vi "UI Producer Consumer-generate-waveform.vi"() -> ()   [LabVIEW 2020]
doc: "This VI illustrates an architecture that allows the user to queue multiple processes. Each process contains multiple state, or in this case stages.The queueing of events is handled by the producer UI loop while the consumer loop goes through each process' states. The processes can have functionality different from one another or can have the same functionality. This architecture allows for expansion on the number of processes as well as the number of states for each process by augmenting the states enum and inputting state functionality in the state case. I have changed the consumer loop to have a time of 500 ms in order to make it easier for the user to enqueue elements. The slowed down consumer loops allowed queue processes to build due to the slow progression of the queue. To hasten the program, the user can change the time constant.\n\nThis type of architecture can apply to an application containing multiple processes, who each have multiple states. This allows the user to easily queue up processes that will proceed in the order that the user selects. There is also two different stop functionalities in order to ensure that a current process is completed or that the current state is completed before stopping the program. This can easily be scaled by editing the type-def enum and adding states to the state machine."
uses:
  States.ctl
panel:
  in  "Output Array":T1(array[cluster])=[{"Waveform Type"=0, "Amplitude"=1.0, "Frequency"=10.0}] {"Frequency" format="%0.2p"; "Amplitude" format="%0.2p"; "Waveform Type" items=["Sine Wave", "Triangle Wave", "Square Wave", "Sawtooth Wave"]}
  in  "Physical Channel(s)":tag="DAQ1/ao0"
  in  "error in (no error)":errorcluster
  out "error out":errorcluster
  in  "Emergency Stop Button":bool
  out "Queue":T2[](array[typedef])
  out "Cluster":T3
  in  "Stop Button":bool
  in  "Process 3":bool
  in  "Process 2":bool
  in  "Process 1":bool
  # "Overview: A producer/consumer architecture with a UI producer loop and a state machine consumer loop. Allows the user to queue multiple state sequences.\nRequirements: LabVIEW 2012 (or compatible\nInstructions:\n1. Run the VI.\n2. Press various Process buttons to see the Queue build.\n3. See the Process and Stage in the Cluster of Boolean indicators.\n4. Press Stop during Process to see Stop functionality.\n5. Run VI again after the program has stopped.\n6. Repeat step 2.\n7. Press Emergency Stop button to see Emergency Stop functionality."
  # "Click the Process button of your choice to enqueue the process of your choice. \nThe Processes will execute in the order that you queue them in."
  # "Stop Button stops program after current process has finished"
  # "Emergency Stop Button stops program after the current state. Press this button to stop in the middle of a Process"
  # "Shows the current Queue."
  # "The Boolean Cluster shows you what process is occurring and the stage it is on.\nEach stage corresponds to a state in a process."
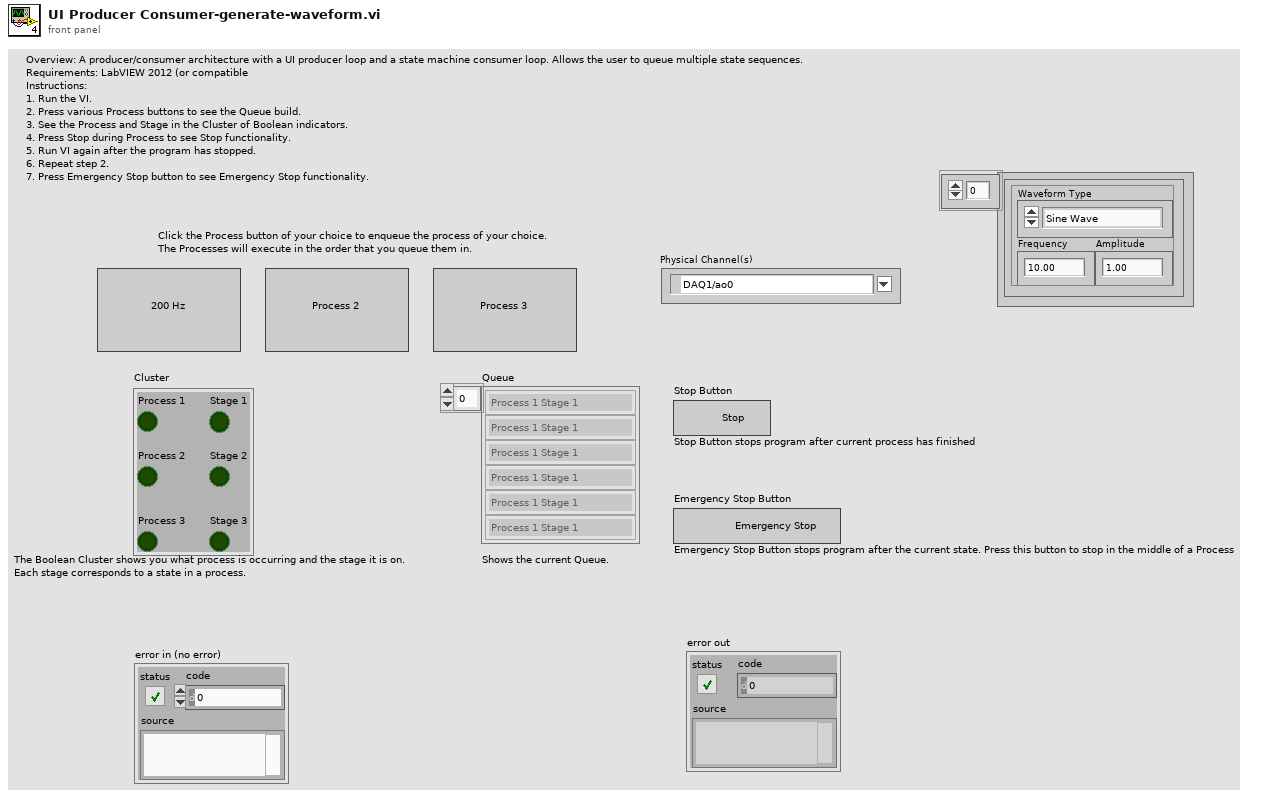
[diagram p1: front panel]
types:
  T1 = cluster{"Waveform Type":u16, "Amplitude":dbl, "Frequency":dbl}[]
  T2 = typedef "States.ctl" = enum16{"Process 1 Stage 1", "Process 1 Stage 2", "Process 1 Stage 3", "Process 2 Stage 1", "Process 2 Stage 2", "Process 2 Stage 3", "Process 3 Stage 1", "Process 3 Stage 2", "Process 3 Stage 3", "Wait", "Stop", "Emergency Stop"}
  T3 = cluster{"Process 1":bool, "Stage 1":bool, "Process 2":bool, "Stage 2":bool, "Process 3":bool, "Stage 3":bool}
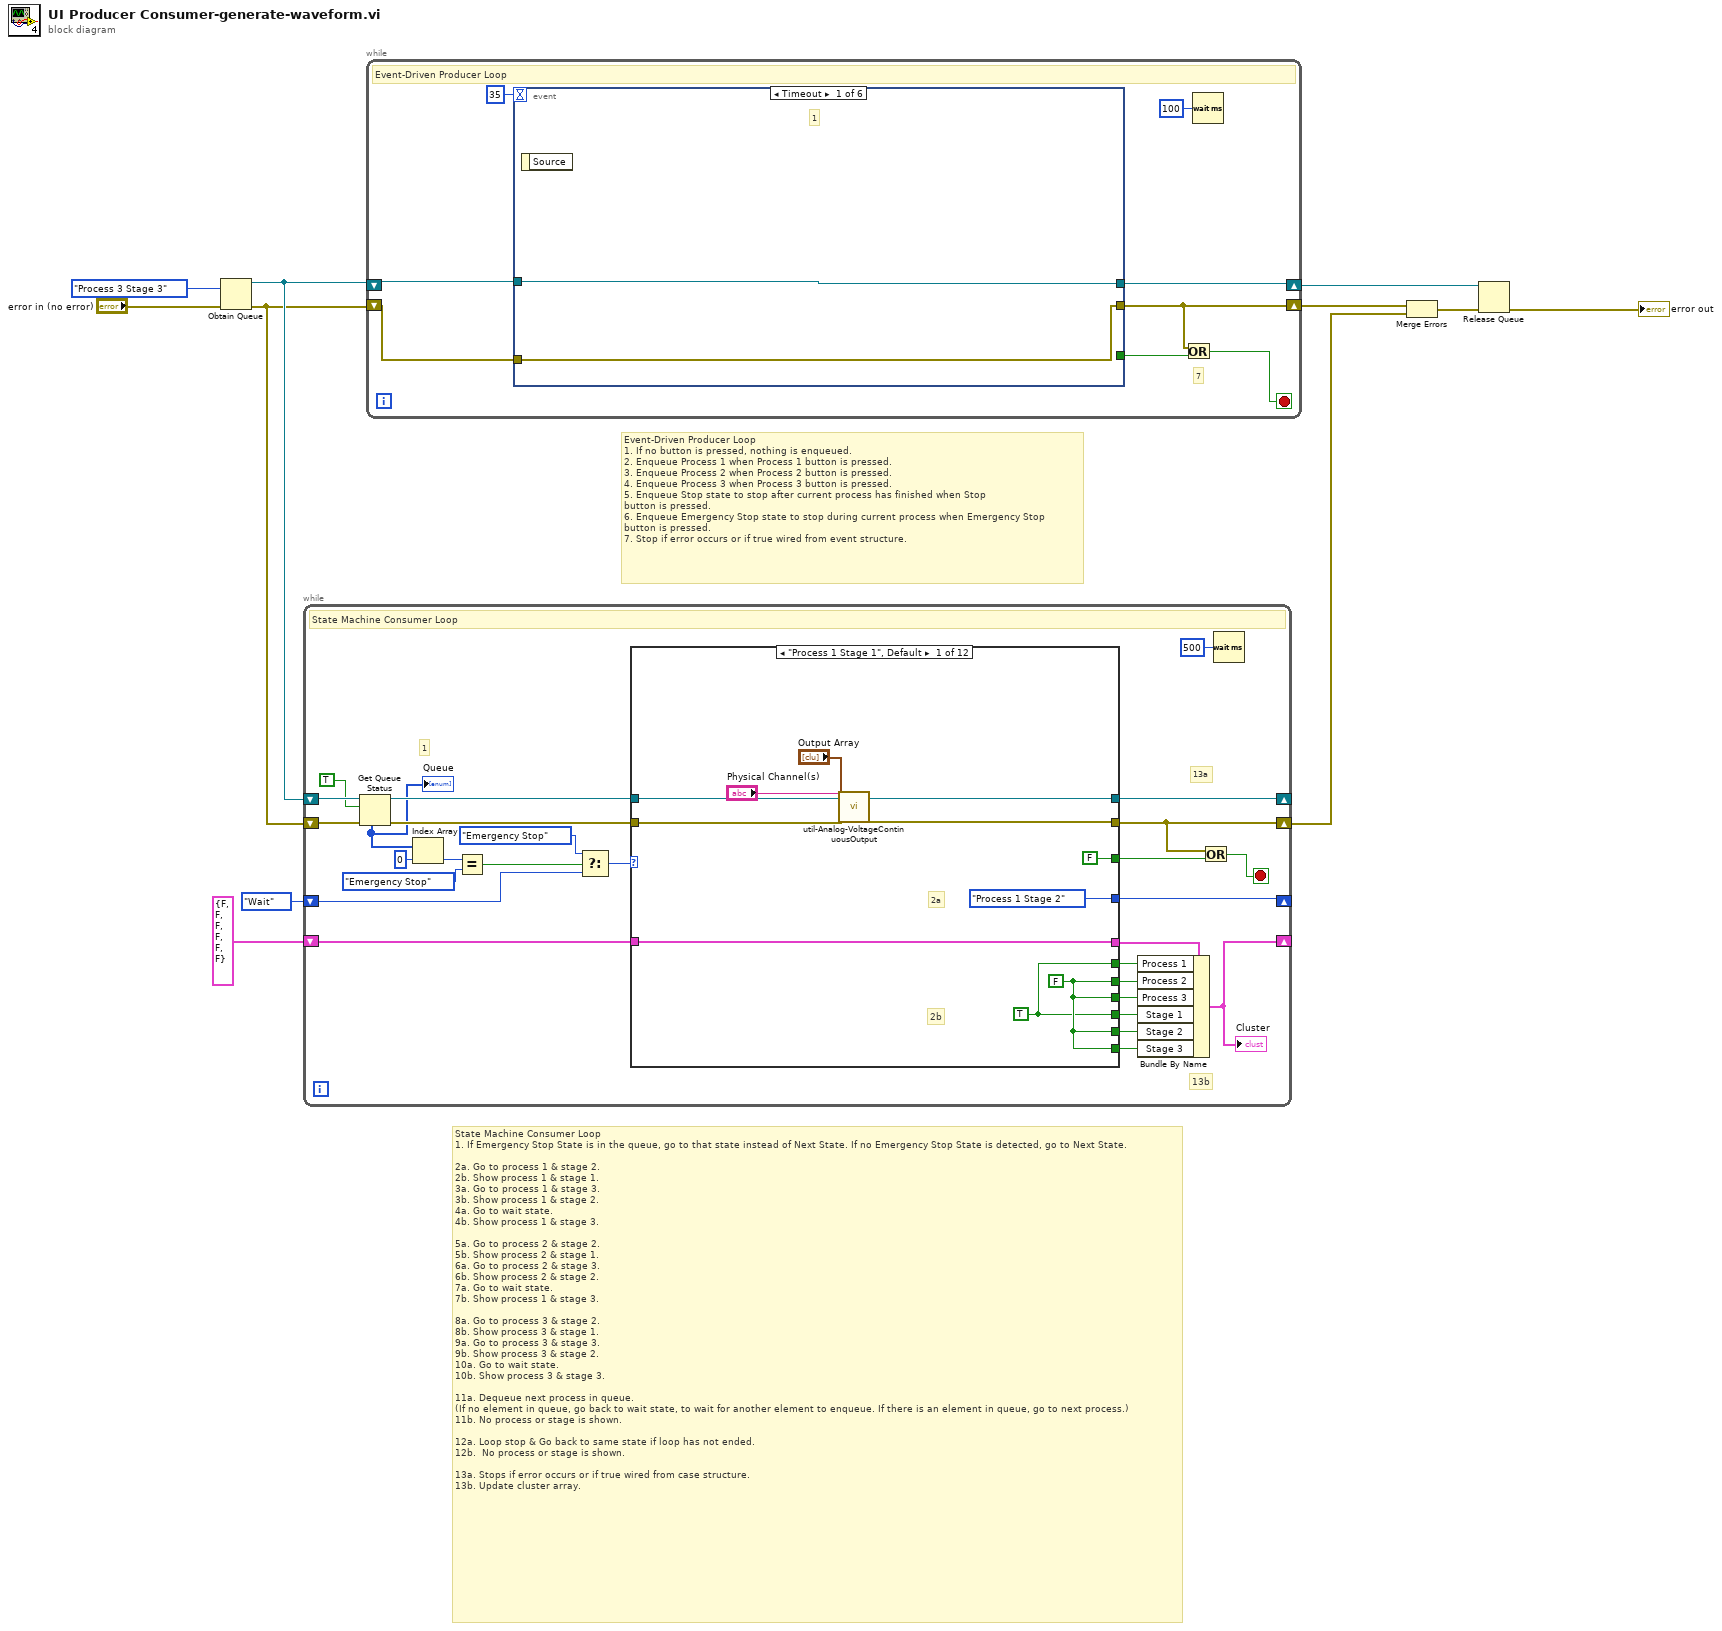
[diagram p0: block diagram]
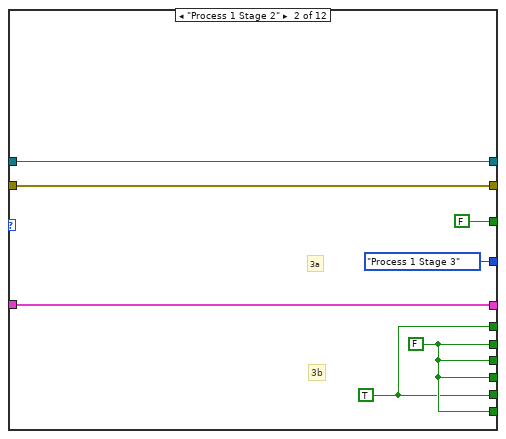
[diagram p2: hidden frame]
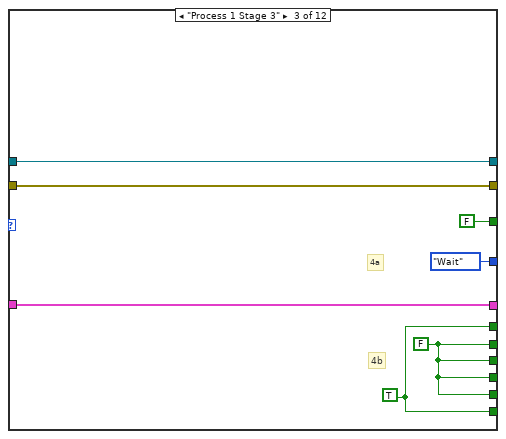
[diagram p3: hidden frame]
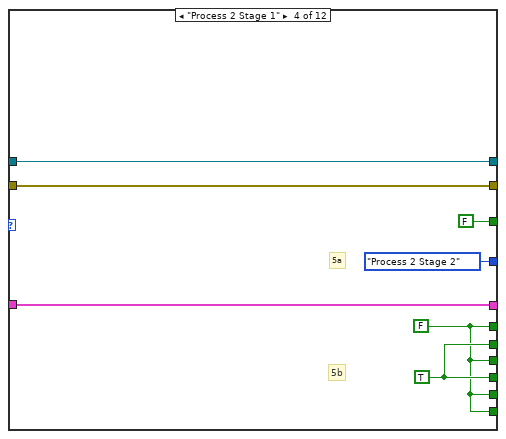
[diagram p4: hidden frame]
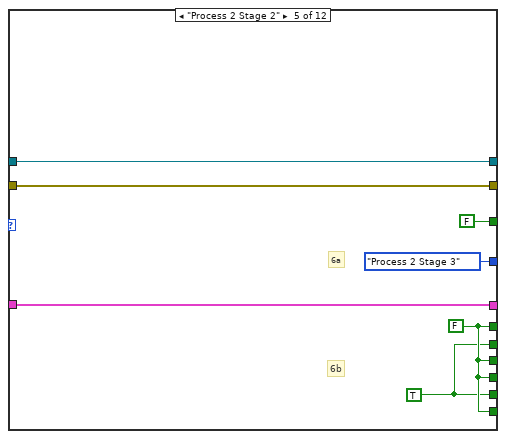
[diagram p5: hidden frame]
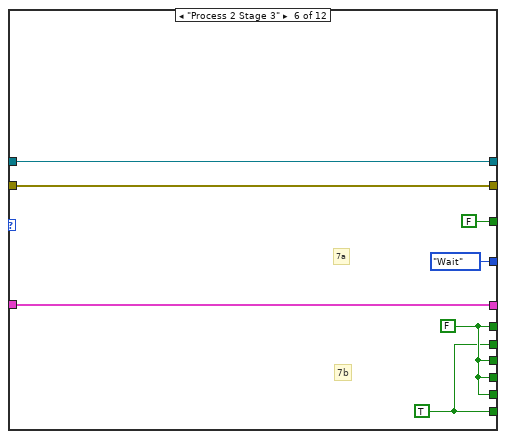
[diagram p6: hidden frame]
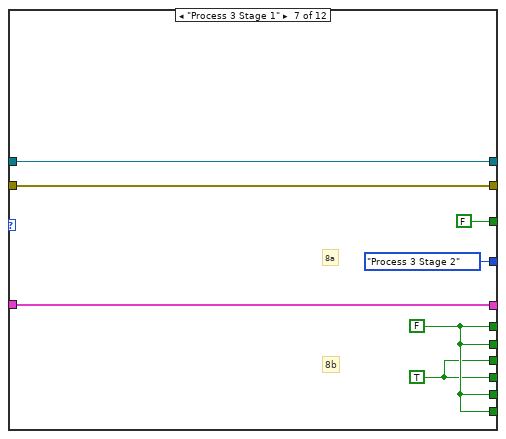
[diagram p7: hidden frame]
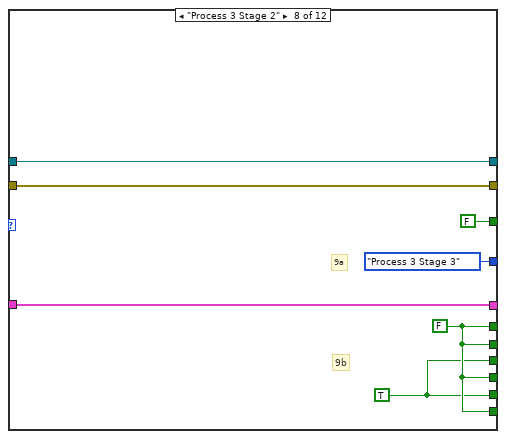
[diagram p8: hidden frame]
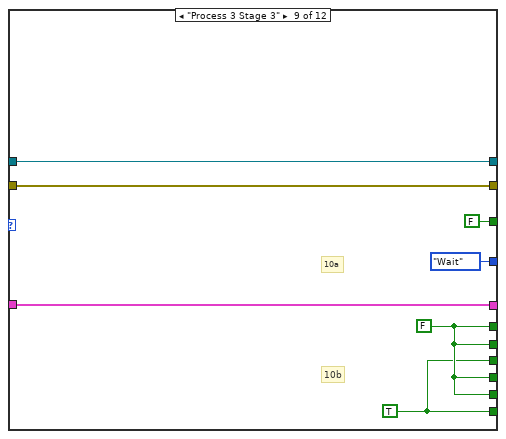
[diagram p9: hidden frame]
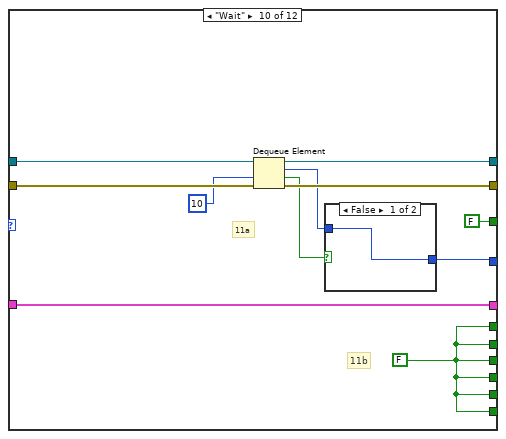
[diagram p10: hidden frame]
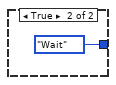
[diagram p11: hidden frame]
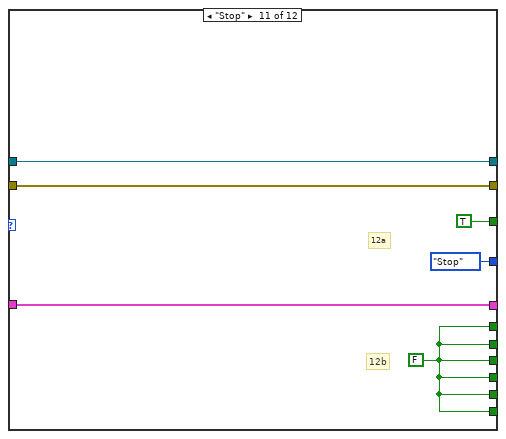
[diagram p12: hidden frame]
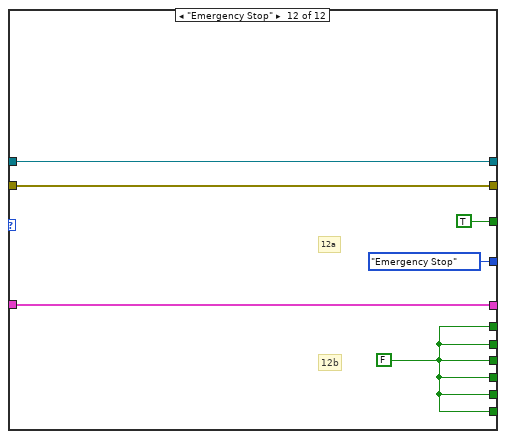
[diagram p13: hidden frame]
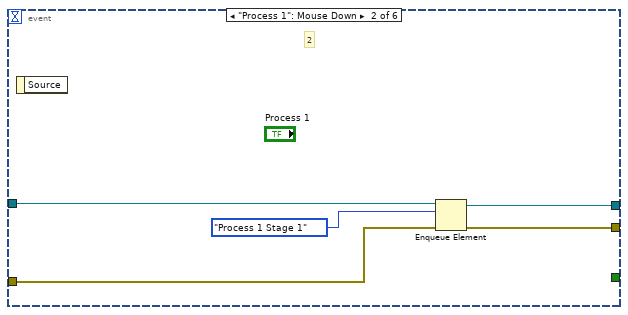
[diagram p14: hidden frame]
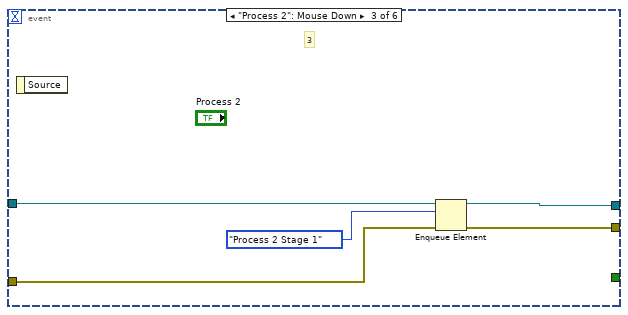
[diagram p15: hidden frame]
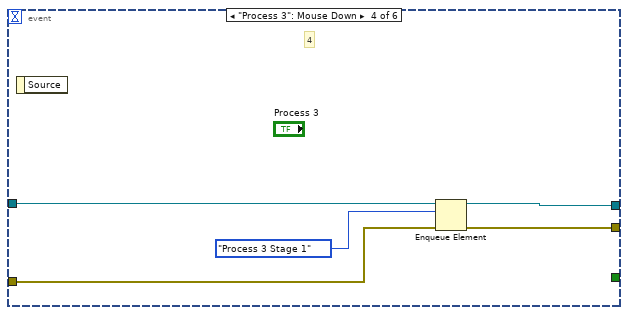
[diagram p16: hidden frame]
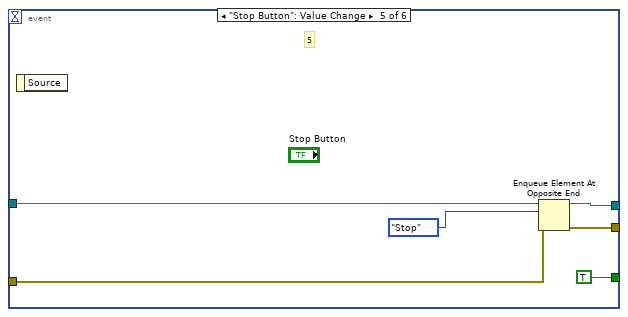
[diagram p17: hidden frame]
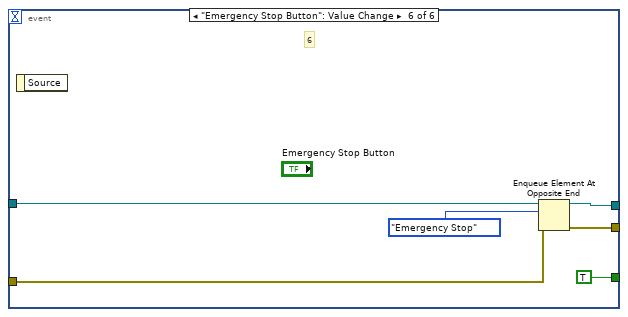
[diagram p18: hidden frame]
diagram:
  # "State Machine Consumer Loop\n1. If Emergency Stop State is in the queue, go to that state instead of Next State. If no Emergency Stop State is detected, go to Next State.\n\n2a. Go to process 1 & stage 2.\n2b. Show process 1 & stage 1.\n3a. Go to process 1 & stage 3.\n3b. Show process 1 & stage 2.\n4a. Go to wait state.\n4b. Show process 1 & stage 3.\n\n5a. Go to process 2 & stage 2.\n5b. Show process 2 & stage 1.\n6a. Go to process 2 & stage 3.\n6b. Show process 2 & stage 2.\n7a. Go to wait state.\n7b. Show process 1 & stage 3.\n\n8a. Go to process 3 & stage 2.\n8b. Show process 3 & stage 1.\n9a. Go to process 3 & stage 3.\n9b. Show process 3 & stage 2.\n10a. Go to wait state.\n10b. Show process 3 & stage 3.\n\n11a. Dequeue next process in queue.\n(If no element in queue, go back to wait state, to wait for another element to enqueue. If there is an element in queue, go to next process.)\n11b. No process or stage is shown.\n\n12a. Loop stop & Go back to same state if loop has not ended.\n12b.  No process or stage is shown.\n\n13a. Stops if error occurs or if true wired from case structure.\n13b. Update cluster array."
  # "Event-Driven Producer Loop\n1. If no button is pressed, nothing is enqueued.\n2. Enqueue Process 1 when Process 1 button is pressed.\n3. Enqueue Process 2 when Process 2 button is pressed.\n4. Enqueue Process 3 when Process 3 button is pressed.\n5. Enqueue Stop state to stop after current process has finished when Stop\nbutton is pressed.\n6. Enqueue Emergency Stop state to stop during current process when Emergency Stop\nbutton is pressed.\n7. Stop if error occurs or if true wired from event structure."
  n1 = Obtain Queue(element data type=States."Process 3 Stage 3", error in (no error)="error in (no error)") -> (queue out=w11:refnum<queue>, error out=w10:errorcluster)  [unwired: 3 in, 1 out]
  n2 = while {
    shift-right: [w25] -> _
    shift-left: w11 -> [w37]
    shift-right: [w21] -> w3
    shift-left: w10 -> [w36]
    shift-right: [w24] -> _
    shift-left: States."Wait" ("y") -> [w14]
    shift-right: [w32] -> _
    shift-left: T3 {"Process 1"=FALSE, "Stage 1"=FALSE, "Process 2"=FALSE, "Stage 2"=FALSE, "Process 3"=FALSE, "Stage 3"=FALSE} ("Cluster") -> [w34]
    stop <- w39 stop-if-true
    # "13a"
    # "13b"
    # "1"
    # "State Machine Consumer Loop"
    n3 = Get Queue Status(queue=w37, return elements? (F)=TRUE, error in (no error)=w36) -> (queue out=w35:refnum<queue>, error out=w22:errorcluster, elements=w19:T2[])  [unwired: 5 out]
    "Queue" <- w19
    n4 = Index Array(array=w19, index=0) -> (element=w17:T2)
    n5 = Equal?(x=w17, y=States."Emergency Stop") -> (x = y?=w15:bool)
    n6 = Select(t=States."Emergency Stop", s=w15, f=w14) -> (s? t:f=w12:T2)
    n7 = case shown="\"Process 1 Stage 1\", Default" w12 {
      tunnel: w35 -> [w46 w53 w62 w69 w76 w83 w90 w97 w104 w114 w124 w130]
      tunnel: w22 -> [w43 w52 w61 w68 w75 w82 w89 w96 w103 w113 w123 w129]
      tunnel: w34 -> [w49 w56 w63 w70 w77 w84 w91 w98 w105 w116 w122 w128]
      tunnel: [w49 w56 w63 w70 w77 w84 w91 w98 w105 w116 w122 w128] -> w33
      tunnel: [w47 w54 w59 w66 w74 w81 w88 w95 w102 w115 w121 w127] -> w31
      tunnel: [w48 w54 w60 w66 w73 w81 w88 w94 w102 w115 w121 w127] -> w30
      tunnel: [w48 w55 w60 w67 w73 w80 w88 w95 w102 w115 w121 w127] -> w29
      tunnel: [w48 w55 w60 w66 w74 w81 w87 w94 w101 w115 w121 w127] -> w28
      tunnel: [w47 w55 w60 w67 w74 w81 w87 w95 w102 w115 w121 w127] -> w27
      tunnel: [w48 w55 w59 w66 w74 w80 w88 w95 w101 w115 w121 w127] -> w26
      tunnel: [w46 w53 w62 w69 w76 w83 w90 w97 w104 w112 w124 w130] -> w25
      tunnel: [w42 w52 w61 w68 w75 w82 w89 w96 w103 w111 w123 w129] -> w21
      tunnel: [States."Process 1 Stage 2" ("y") States."Process 1 Stage 3" ("y") States."Wait" ("y") States."Process 2 Stage 2" ("y") States."Process 2 Stage 3" ("y") States."Wait" ("y") States."Process 3 Stage 2" ("y") States."Process 3 Stage 3" ("y") States."Wait" ("y") w108 States."Stop" ("y") States."Emergency Stop" ("y")] -> w24
      tunnel: [FALSE FALSE FALSE FALSE FALSE FALSE FALSE FALSE FALSE FALSE TRUE TRUE] -> w23
      frame "Process 1 Stage 1", Default {
        w47 = TRUE
        w48 = FALSE
        # "2b"
        # "2a"
        n8 = call "util-Analog-VoltageContinuousOutput.vi"("Channel(s)"="Physical Channel(s)", "Output Array"="Output Array", "error in"=w43) -> ("error out"=w42:errorcluster)  [unwired: 23 in, 1 out]
      }
      frame "Process 1 Stage 2" {
        w55 = FALSE
        w54 = TRUE
        # "3b"
        # "3a"
      }
      frame "Process 1 Stage 3" {
        w60 = FALSE
        w59 = TRUE
        # "4b"
        # "4a"
      }
      frame "Process 2 Stage 1" {
        w66 = FALSE
        w67 = TRUE
        # "5b"
        # "5a"
      }
      frame "Process 2 Stage 2" {
        w74 = FALSE
        w73 = TRUE
        # "6a"
        # "6b"
      }
      frame "Process 2 Stage 3" {
        w81 = FALSE
        w80 = TRUE
        # "7a"
        # "7b"
      }
      frame "Process 3 Stage 1" {
        w88 = FALSE
        w87 = TRUE
        # "8b"
        # "8a"
      }
      frame "Process 3 Stage 2" {
        w95 = FALSE
        w94 = TRUE
        # "9a"
        # "9b"
      }
      frame "Process 3 Stage 3" {
        w102 = FALSE
        w101 = TRUE
        # "10a"
        # "10b"
      }
      frame "Wait" {
        w115 = FALSE
        # "11b"
        # "11a"
        n9 = Dequeue Element(queue=w114, timeout in ms (-1)=10, error in (no error)=w113) -> (queue out=w112:refnum<queue>, element=w109:T2, timed out?=w110:bool, error out=w111:errorcluster)
        n10 = case shown="False" w110 {
          tunnel: w109 -> [w117 _]
          tunnel: [w117 States."Wait" ("y")] -> w108
          frame False {
          }
          frame True {
          }
        }
      }
      frame "Stop" {
        w121 = FALSE
        # "12a"
        # "12b"
      }
      frame "Emergency Stop" {
        w127 = FALSE
        # "12b"
        # "12a"
      }
    }
    n11 = Bundle By Name(cluster=w33, "Process 1"=w31, "Process 2"=w29, "Process 3"=w28, "Stage 1"=w27, "Stage 2"=w30, "Stage 3"=w26) -> (w32:T3)
    "Cluster" <- w32
    n12 = Or(x=w21, y=w23) -> (x .or. y?=w39:bool)
    n13 = Wait (ms)(milliseconds to wait=u32 500) -> ()  [unwired: 1 out]
  }
  n14 = while {
    shift-right: [w135] -> w7
    shift-left: w11 -> [w137]
    shift-right: [w134] -> w9
    shift-left: w10 -> [w136]
    stop <- w132 stop-if-true
    # "7"
    # "Event-Driven Producer Loop"
    n15 = event shown="[0] Timeout" {
      selector: _ -> [_ _ _ _ _ _]
      dyn-events: _ -> [_ _ _ _ _ _]
      timeout: 35 -> [_ _ _ _ _ _]
      tunnel: w137 -> [w140 w145 w150 w155 w161 w167]
      tunnel: w136 -> [w139 w143 w148 w153 w160 w166]
      tunnel: [w139 w142 w147 w152 w158 w164] -> w134
      tunnel: [w140 w144 w149 w154 w159 w165] -> w135
      tunnel: [_ _ _ _ TRUE TRUE] -> w133
      event Timeout {
        # "1"
        n16 = event-data() -> ()  [unwired: 1 in, 1 out]
      }
      event "Process 1": Mouse Down {
        # "2"
        n17 = event-data() -> ()  [unwired: 1 in, 1 out]
        n18 = Enqueue Element(queue=w145, element=States."Process 1 Stage 1", error in (no error)=w143) -> (queue out=w144:refnum<queue>, error out=w142:errorcluster)  [unwired: 1 in, 1 out]
      }
      event "Process 2": Mouse Down {
        # "3"
        n19 = event-data() -> ()  [unwired: 1 in, 1 out]
        n20 = Enqueue Element(queue=w150, element=States."Process 2 Stage 1", error in (no error)=w148) -> (queue out=w149:refnum<queue>, error out=w147:errorcluster)  [unwired: 1 in, 1 out]
      }
      event "Process 3": Mouse Down {
        # "4"
        n21 = event-data() -> ()  [unwired: 1 in, 1 out]
        n22 = Enqueue Element(queue=w155, element=States."Process 3 Stage 1", error in (no error)=w153) -> (queue out=w154:refnum<queue>, error out=w152:errorcluster)  [unwired: 1 in, 1 out]
      }
      event "Stop Button": Value Change {
        # "5"
        n23 = event-data() -> ()  [unwired: 1 in, 1 out]
        n24 = Enqueue Element At Opposite End(queue=w161, element=States."Stop", error in (no error)=w160) -> (queue out=w159:refnum<queue>, error out=w158:errorcluster)  [unwired: 1 in, 1 out]
      }
      event "Emergency Stop Button": Value Change {
        # "6"
        n25 = event-data() -> ()  [unwired: 1 in, 1 out]
        n26 = Enqueue Element At Opposite End(queue=w167, element=States."Emergency Stop", error in (no error)=w166) -> (queue out=w165:refnum<queue>, error out=w164:errorcluster)  [unwired: 1 in, 1 out]
      }
    }
    n27 = Or(x=w134, y=w133) -> (x .or. y?=w132:bool)
    n28 = Wait (ms)(milliseconds to wait=u32 100) -> ()  [unwired: 1 out]
  }
  n29 = Merge Errors(w9, w3) -> (w8:errorcluster)
  n30 = Release Queue(queue=w7, error in (no error)=w8) -> (error out=→"error out":errorcluster)  [unwired: 1 in, 2 out]
